vi "samples write (host).vi"(6 "trigger to write samples":bool, 7 "samples num":u32=1000, 9 "number of packets to detect":u32, 10 "file for writing samples":refnum<file>, 11 "fpga cluster":T1 {"Daughterboard Clock Rate" format="%#.3pHz"; "FPGA Data Clock Rate" format="%#.3pHz"; "Data Clock Rate" format="%#.3pHz"; "Characterization Data"."Frequencies [Hz]" format="%#_6p"; "EEPROM Characterization Header"."Pointer to Device Data Header" format="%x"; "EEPROM Characterization Header"."Checksum" format="%x"; "Device Data Header"."Pointer to Characterization Data" format="%x"; "Device Data Header"."Checksum" format="%x"; "EEPROM Header"."Pointer to User Header" format="%x"; "EEPROM Header"."Pointer to Factory Header" format="%x"; "EEPROM Header"."Product Code" format="%x"; "EEPROM Header"."Checksum" format="%x"}) -> (1 "samples num":u32, 2 "samples is written":bool, 3 "samples":string)   [LabVIEW 2020]
uses:
  <instrlib>/niUsrpRio/Config/v1/Host/Public/niUsrpRio Session.ctl
  <instrlib>/_niInstr/Register Bus/v0/Host/Public/Register Bus Session.ctl
  <instrlib>/_niInstr/Register Bus/v0/Host/Private/Session Data.ctl
  <instrlib>/niUsrpRio/Config/v1/Host/Private/DB Queue Reference.ctl
  <instrlib>/niUsrpRio/Config/v1/Host/Private/Daughterboard Data.ctl
  <instrlib>/niUsrpRio/Config/v1/Host/Private/ATR state data.ctl
  <instrlib>/niUsrpRio/Config/v1/Host/Private/Antenna Configuration.ctl
  <instrlib>/niUsrpRio/Config/v1/Host/Private/CPLD Power Mode.ctl
  <instrlib>/niUsrpRio/Config/v1/Host/Public/EEPROM Header.ctl
  <instrlib>/niUsrpRio/Config/v1/Host/Public/EEPROM Device Data Header.ctl
  <instrlib>/niUsrpRio/Config/v1/Host/Public/EEPROM Characterization Header.ctl
  <instrlib>/niUsrpRio/Config/v1/Host/Public/Characterization Data.ctl
  <instrlib>/niUsrpRio/Config/v1/Host/Public/IQ Imbalance.ctl
  Host/SubVIs/Streaming Xvcr FPGA Ref.ctl
  <vilib>/Utility/error.llb/Error Cluster From Error Code.vi
  <vilib>/rvi/errors/niLvFpgaAdjustHostInterfaceError.vi
  <vilib>/rvi/interface/nirviMethod/nirviMethod.xnode
  <vilib>/rvi/errors/niLvFpgaMergeErrorWithErrorCode.vi
  <vilib>/FPGAPlugInAG/Dynamic/niLvFpga_ReadFifo_Dynamic.vi
  <vilib>/FPGAPlugInAG/Dynamic/niLvFpga_ConfigureFifo_Dynamic.vi
  <instrlib>/_niInstr/Register Bus/v0/Host/niInstr Register Bus v0 Host.lvlib
  <instrlib>/niUsrpRio/Config/v1/Host/niUsrpRio Config v1 Host.lvlib
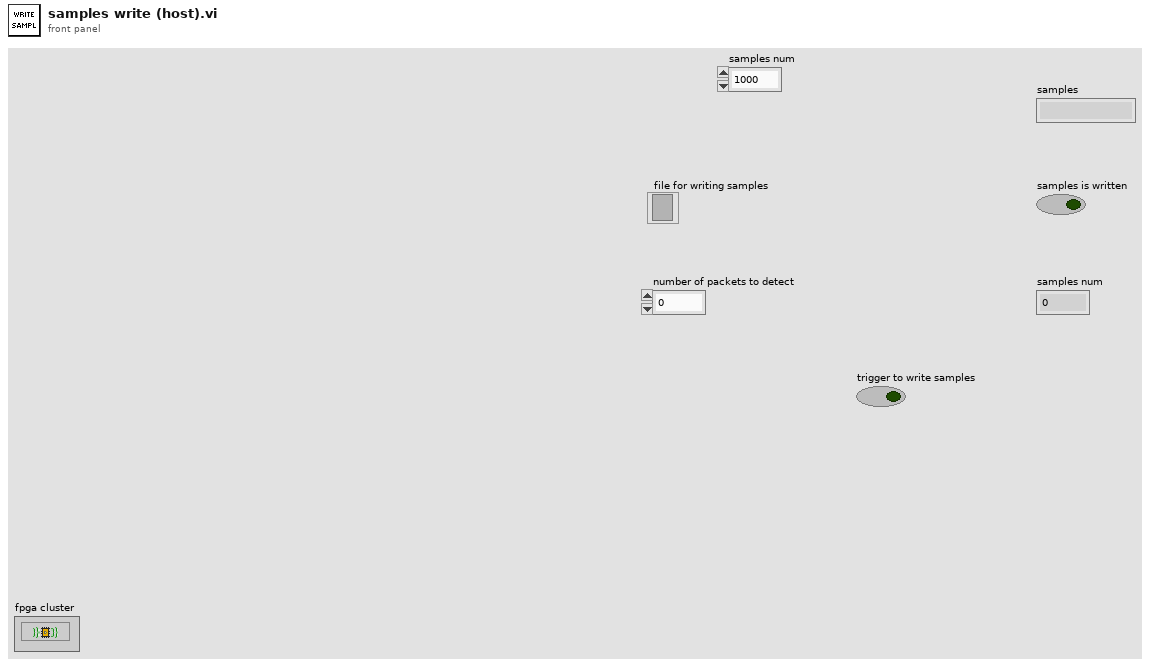
[diagram p1: front panel]
types:
  T1 = typedef "niUsrpRio Config v1 Host.lvlib/niUsrpRio Session.ctl" = cluster{"FPGA Interface":refnum<k20>, "RIO Interface Number":u32, "Data Clock Rate":u32, "FPGA Data Clock Rate":u32, "Global Settings Register Bus":T2, "Radio 0 Settings Register Bus":T2, "Radio 1 Settings Register Bus":T2, "Radio Settings Bus Semaphore":T3, "DB Queues":T4[], "Characterization Data Valid?":bool, "EEPROM Header":T5, "Device Data Header":T6, "EEPROM Characterization Header":T7, "Characterization Data":T8[], "FPGA Current Version":u32, "FPGA Oldest Compatible Version":u32, "Fixed Logic Current Version":u32, "Fixed Logic Oldest Compatible Version":u32, "FPGA Radio Settings Bus Current Version":u32, "FPGA Radio Settings Bus Oldest Compatible Version":u32, "FPGA Board Config Current Version":u32, "FPGA Board Config Oldest Compatible Version":u32, "Daughterboard Clock Rate":u32, "daughterboard configuration session handles":u64[]}
  T2 = typedef "niInstr Register Bus v0 Host.lvlib/Register Bus Session.ctl" = refnum<queue>
  T3 = typedef "Semaphore RefNum" = refnum<k1>
  T4 = typedef "niUsrpRio Config v1 Host.lvlib/DB Queue Reference.ctl" = refnum<queue>
  T5 = typedef "niUsrpRio Config v1 Host.lvlib/EEPROM Header.ctl" = cluster{"Checksum":u32, "Product Code":u16, "Hardware Current Version":u16, "Hardware Oldest Compatible Version":u16, "EEPROM Map Current Version":u16, "EEPROM Map Oldest Compatible Version":u16, "User Password":string, "Pointer to Factory Header":u32, "Pointer to User Header":u32, "Recommended Interval":u16, "Number of Reserved Bytes":i32, "Number of Daughterboards":u8, "Daughterboard IDs":u16[], "Daughterboard Serial Numbers":string[]}
  T6 = typedef "niUsrpRio Config v1 Host.lvlib/EEPROM Device Data Header.ctl" = cluster{"Checksum":u32, "Number of Channels":u8, "Number of Gain Settings":u16[], "Pointer to Characterization Data":u32[], "Number of Reserved Bytes":i32, "Number of Frequencies":u16[]}
  T7 = typedef "niUsrpRio Config v1 Host.lvlib/EEPROM Characterization Header.ctl" = cluster{"Checksum":u32, "Date":timestamp, "Temperature":sgl, "Misc. Info":string, "Pointer to Device Data Header":u32, "Number of Reserved Bytes":i32}
  T8 = typedef "niUsrpRio Config v1 Host.lvlib/Characterization Data.ctl" = cluster{"Gains[dB]":dbl[], "Frequencies [Hz]":dbl[], "IQ Imbalance Table":T9[], "Measured Gains[dB]":dbl[][]}
  T9 = typedef "niUsrpRio Config v1 Host.lvlib/IQ Imbalance.ctl" = cluster{"Gain Imbalance [linear]":dbl, "Phase Imbalance [radians]":dbl, "Offset":cdb}
  T10 = typedef "Streaming Xvcr FPGA Ref.ctl" = refnum<k20>
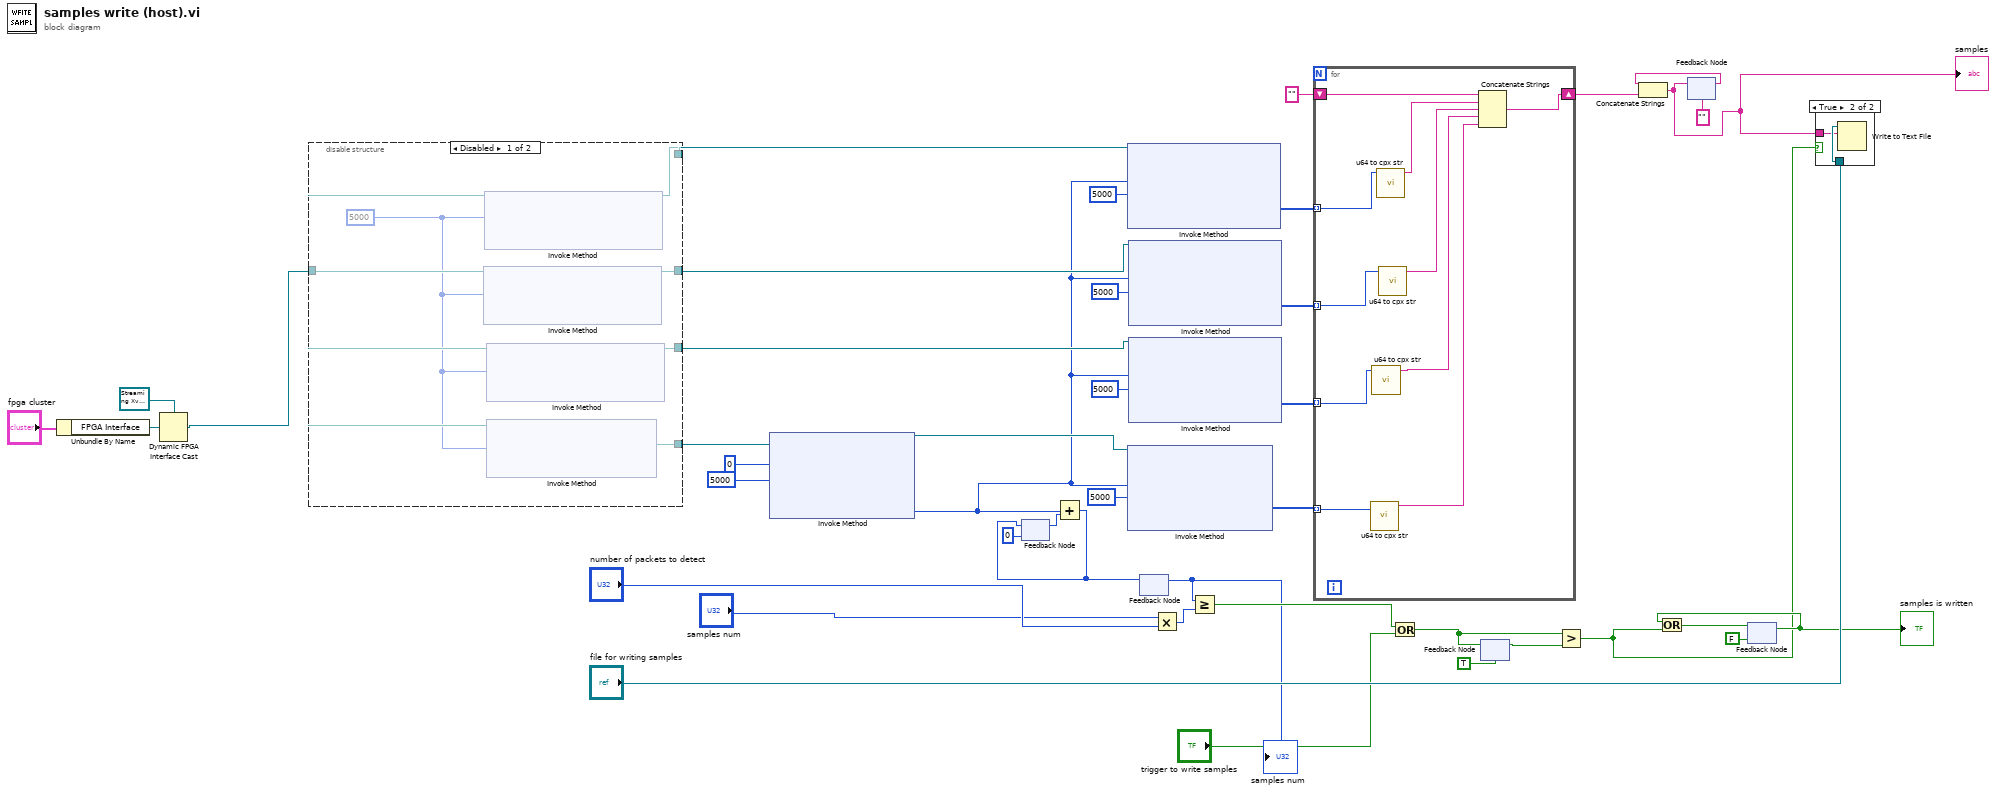
[diagram p0: block diagram]
diagram:
  n1 = Unbundle By Name("fpga cluster") -> ("FPGA Interface"=w6:refnum<k20>)
  n2 = Dynamic FPGA Interface Cast(Session In=T10 refnum ("Type"), Type=w6) -> (Session Out=w3:T10)
  n3 = disable-structure shown="Disabled" {
    disable-tunnel: [w48 w49] -> w16
    disable-tunnel: [w47 w49] -> w12
    disable-tunnel: [w46 w49] -> w11
    disable-tunnel: [w45 w49] -> w10
    disable-tunnel: w3 -> [w44 w49]
    frame Disabled {
      w43 = u32 5000 ("Requested Depth")
      n4 = xnode "Invoke Method"("FPGA VI Reference In"=w44, "Requested Depth"=w43) -> ("FPGA VI Reference Out"=w46:T10)  [unwired: 1 in, 2 out]
      n5 = xnode "Invoke Method"("FPGA VI Reference In"=w44, "Requested Depth"=w43) -> ("FPGA VI Reference Out"=w47:T10)  [unwired: 1 in, 2 out]
      n6 = xnode "Invoke Method"("FPGA VI Reference In"=w44, "Requested Depth"=w43) -> ("FPGA VI Reference Out"=w45:T10)  [unwired: 1 in, 2 out]
      n7 = xnode "Invoke Method"("FPGA VI Reference In"=w44, "Requested Depth"=w43) -> ("FPGA VI Reference Out"=w48:T10)  [unwired: 1 in, 2 out]
    }
    frame Enabled {
    }
  }
  n8 = xnode "Invoke Method"("FPGA VI Reference In"=w16, "Number of Elements"=u32 0, "Timeout (ms)"=5000) -> ("FPGA VI Reference Out"=w25:T10, "Elements Remaining"=w1:u32)  [unwired: 1 in, 2 out]
  n9 = feedback #1(u32 0) -> (w29:u32)
  n10 = Add(x=w1, y=w29) -> (x+y=w31:u32)
  n11 = feedback-in #1(w31) -> ()
  n12 = xnode "Invoke Method"("FPGA VI Reference In"=w12, "Number of Elements"=w1, "Timeout (ms)"=5000) -> ("Data"=w9:u64[])  [unwired: 1 in, 3 out]
  n13 = xnode "Invoke Method"("FPGA VI Reference In"=w25, "Number of Elements"=w1, "Timeout (ms)"=5000) -> ("Data"=w23:u64[])  [unwired: 1 in, 3 out]
  n14 = xnode "Invoke Method"("FPGA VI Reference In"=w11, "Number of Elements"=w1, "Timeout (ms)"=5000) -> ("Data"=w8:u64[])  [unwired: 1 in, 3 out]
  n15 = xnode "Invoke Method"("FPGA VI Reference In"=w10, "Number of Elements"=w1, "Timeout (ms)"=5000) -> ("Data"=w7:u64[])  [unwired: 1 in, 3 out]
  n16 = feedback #2() -> (w35:u32)  [unwired: 1 in]
  "samples num" <- w35
  n17 = feedback-in #2(w31) -> ()
  n18 = Multiply(x="samples num", y="number of packets to detect") -> (x*y=w34:u32)
  n19 = Greater Or Equal?(x=w35, y=w34) -> (x >= y?=w37:bool)
  n20 = for {
    tunnel: w23 -> [w59] mode=indexing
    shift-right: [w50] -> w24
    shift-left: "" -> [w58]
    tunnel: w9 -> [w57] mode=indexing
    tunnel: w8 -> [w56] mode=indexing
    tunnel: w7 -> [w55] mode=indexing
    n21 = call "u64 to cpx str.vi"("Numeric"=w59) -> ("String"=w51:string)  [unwired: 10 in]
    n22 = call "u64 to cpx str.vi"("Numeric"=w55) -> ("String"=w52:string)  [unwired: 10 in]
    n23 = call "u64 to cpx str.vi"("Numeric"=w57) -> ("String"=w54:string)  [unwired: 10 in]
    n24 = call "u64 to cpx str.vi"("Numeric"=w56) -> ("String"=w53:string)  [unwired: 10 in]
    n25 = Concatenate Strings(w58, w54, w53, w52, w51) -> (w50:string)
  }
  n26 = Or(x=w37, y="trigger to write samples") -> (x .or. y?=w33:bool)
  n27 = feedback #3(TRUE ("trigger to write csi and samples")) -> (w27:bool)
  n28 = feedback-in #3(w33) -> ()
  n29 = Greater?(x=w33, y=w27) -> (0:w40:bool)
  n30 = feedback #4("" ("output string")) -> (w21:string)
  n31 = Concatenate Strings(w21, w24) -> (w22:string)
  "samples" <- w22
  n32 = feedback-in #4(w22) -> ()
  n33 = feedback #5(FALSE) -> (w41:bool)
  "samples is written" <- w41
  n34 = Or(x=w41, y=w40) -> (x .or. y?=w39:bool)
  n35 = feedback-in #5(w39) -> ()
  n36 = case shown="True" w40 {
    tunnel: "file for writing samples" -> [_ w61]
    tunnel: w22 -> [_ w60]
    frame False {
    }
    frame True {
      n37 = Write to Text File(file (use dialog)=w61, text=w60) -> ()  [unwired: 2 in, 3 out]
    }
  }
